vi "Vector - set velocity XY.vi"(8 "error in (no error)":errorcluster, 9 "y vel":dbl, 10 "x vel":dbl, 11 "ASI stage":T1) -> (0 "error out":errorcluster)   [LabVIEW 2010]
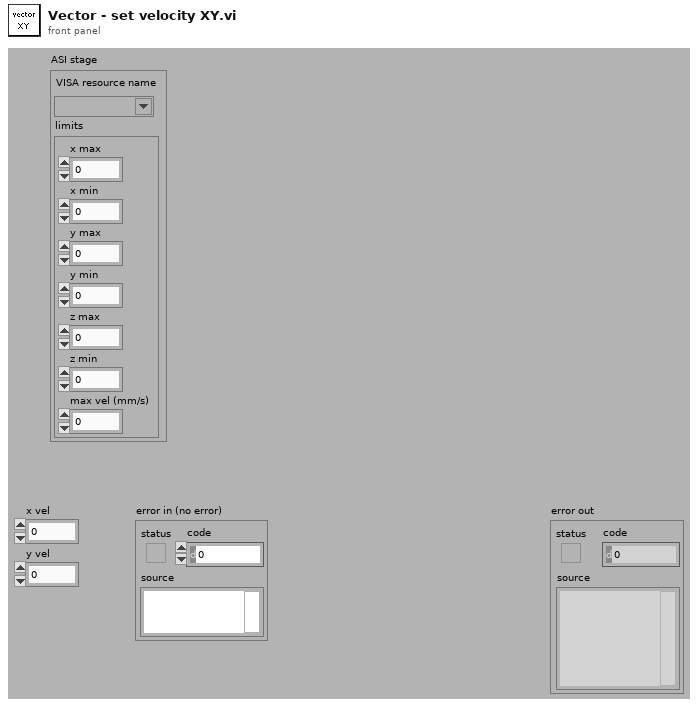
[diagram p1: front panel]
types:
  T1 = cluster{"VISA resource name":refnum<visa-resource-name>, "limits":cluster{"x max":dbl, "x min":dbl, "y max":dbl, "y min":dbl, "z max":dbl, "z min":dbl, "max vel (mm/s)":dbl}}
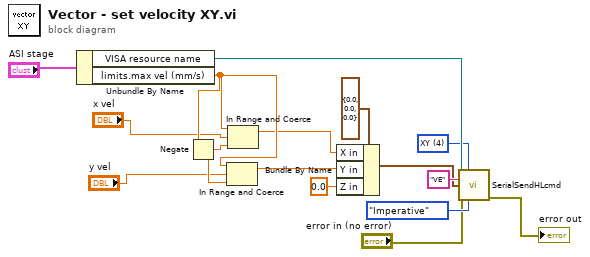
[diagram p0: block diagram]
diagram:
  w14 = u16 4 items=["No axis", "X", "Y", "Z", "XY", "XYZ"] ("Axis configuration")
  n1 = Unbundle By Name("ASI stage") -> ("VISA resource name"=w15:refnum<visa-resource-name>, "limits.max vel (mm/s)"=w8:dbl)
  n2 = Negate(x=w8) -> (-x=w7:dbl)
  n3 = In Range and Coerce(upper limit=w8, x="y vel", lower limit=w7) -> (coerced(x)=w4:dbl)  [unwired: 1 out]
  n4 = In Range and Coerce(upper limit=w8, x="x vel", lower limit=w7) -> (coerced(x)=w3:dbl)  [unwired: 1 out]
  n5 = Bundle By Name(cluster=cluster{"X in":dbl, "Y in":dbl, "Z in":dbl} {"X in"=0.0, "Y in"=0.0, "Z in"=0.0} ("data in"), "X in"=w3, "Y in"=w4, "Z in"=0.0) -> (w2:cluster{"X in":dbl, "Y in":dbl, "Z in":dbl})
  n6 = call "SerialSendHLcmd.vi"("VISA resource name"=w15, "Axis configuration"=w14, "Command"="VE", "data in"=w2, "error in (no error)"="error in (no error)", "Command type"=enum16{"Query", "Where", "Imperative", "DU Y"}."Imperative") -> ("error out"=→"error out":errorcluster)  [unwired: 7 in, 2 out]
